vi "Read Topology Defined Channels.vi"(8 "error in":errorcluster, 11 "2525 in":refnum<class "2525.lvclass">) -> (0 "error out":errorcluster, 3 "2525 out":refnum<class "2525.lvclass">)   [LabVIEW 2019, in "2525.lvlib" / "2525.lvclass"]
uses:
  Library/2525.lvclass
  Library/2525.lvclass/2525.ctl
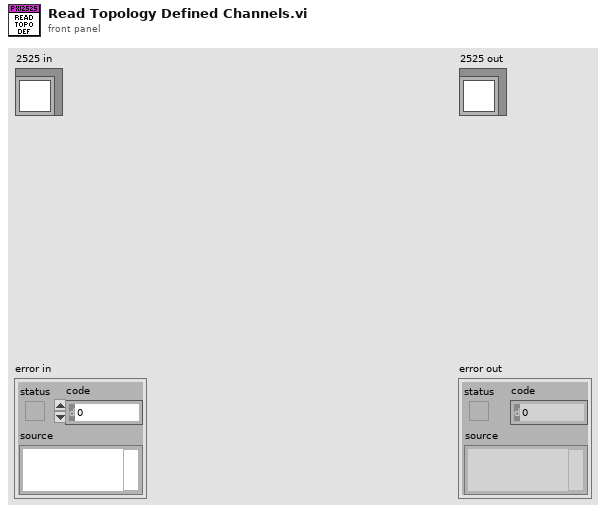
[diagram p1: front panel]
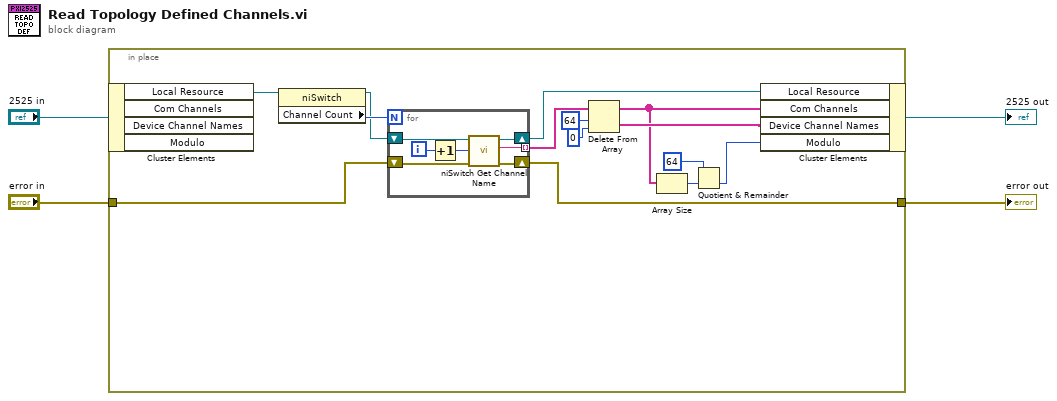
[diagram p0: block diagram]
diagram:
  n1 = in-place {
    in-place-border: "error in" -> [w14]
    in-place-border: [w13] -> w1
    n2 = in-place-cluster #1("2525 in") -> ("Local Resource"=w18:refnum<k15>)  [unwired: 3 out]
    n3 = property class="niSwitch"(reference=w18) -> (reference out=w16:refnum<k15>, "Channel Count"=w17:i32)  [unwired: 1 in, 1 out]
    n4 = for {
      N: w17 -> [_]
      shift-right: [w24] -> w15
      shift-left: w16 -> [w25]
      tunnel: [w23] -> w10 mode=indexing
      shift-right: [w21] -> w13
      shift-left: w14 -> [w22]
      i -> [w20]
      n5 = Increment(x=w20) -> (x+1=w19:i32)
      n6 = call <instrlib>:"niSwitch Get Channel Name.vi"("error in (no error)"=w22, "index (1)"=w19, "instrument handle"=w25) -> ("error out"=w21:errorcluster, "channel string"=w23:string, "instrument handle out"=w24:refnum<k15>)  [unwired: 6 in]
    }
    n7 = Delete From Array(array=w10, length=64, index=0) -> (deleted portion=w9:string[], array with subset deleted=w8:string[])
    n8 = Array Size(array=w8) -> (size(s)=w7:i32)
    n9 = Quotient & Remainder(x=64, y=w7) -> (floor(x/y)=w5:i32)  [unwired: 1 out]
    n10 = in-place-cluster #1("Local Resource"=w15, "Com Channels"=w8, "Device Channel Names"=w9, "Modulo"=w5) -> (→"2525 out":refnum<class "2525.lvclass">)
  }
  "error out" <- w1
